vi "Set Timing.vi"(8 "error in (no error)":errorcluster, 9 "Timing Engine":T1=enum."Low Speed", 10 "TimingCfg":T2, 11 "Chassis Cfg":refnum<class "ChassisCfg.lvclass">) -> (0 "error out":errorcluster, 3 "Chassis Cfg":refnum<class "ChassisCfg.lvclass">)   [LabVIEW 2018, in "Configuration Grandmaster.lvlib" / "ChassisCfg.lvclass"]
uses:
  ChassisCfg.lvclass
  Common/Controls/Group Timing Info.ctl
  Common/Controls/TE_Designator.ctl
  ChassisCfg.lvclass/ChassisCfg.ctl
  Class Timing Group/TimingGrp.lvclass
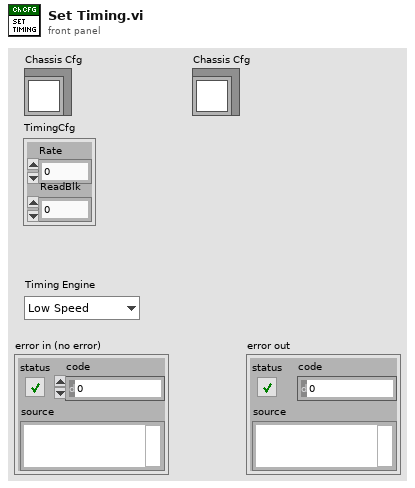
[diagram p1: front panel]
types:
  T1 = typedef "TE_Designator.ctl" = enum16{"High Speed", "Low Speed"}
  T2 = typedef "Group Timing Info.ctl" = cluster{"Rate":dbl, "ReadBlk":i32}
  T3 = typedef "LS Lock Sizes.ctl" = enum16{"No", "250ms", "500ms", "1s"}
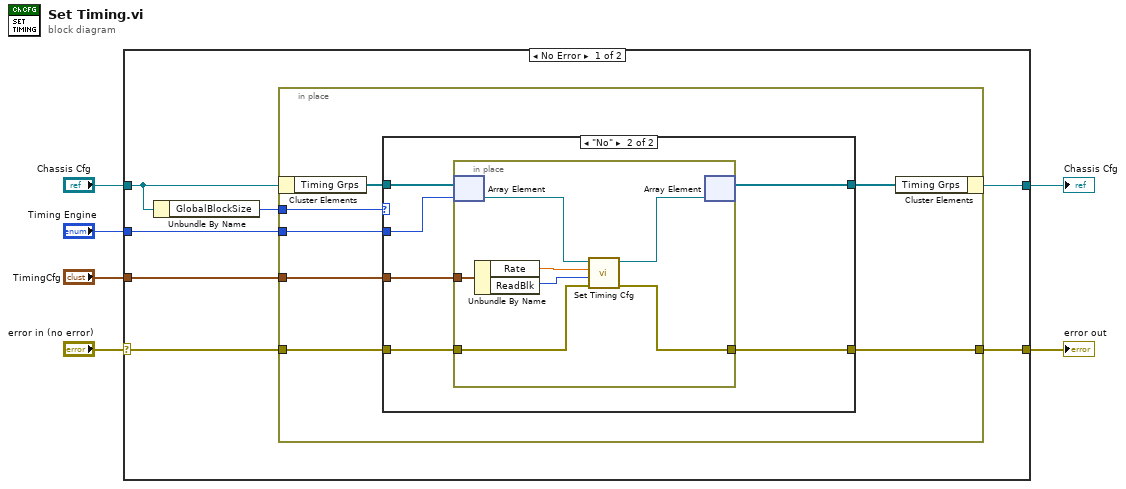
[diagram p0: block diagram]
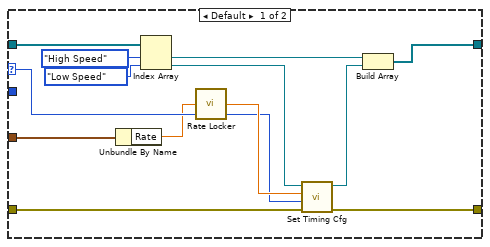
[diagram p2: hidden frame]
diagram:
  n1 = case shown="No Error" "error in (no error)" {
    selector: "error in (no error)" -> [w7 w48]
    tunnel: "TimingCfg" -> [w13 _]
    tunnel: "Timing Engine" -> [w12 _]
    tunnel: [w11 w48] -> w4
    tunnel: [w10 w49] -> w3
    tunnel: "Chassis Cfg" -> [w9 w49]
    frame No Error {
      n2 = Unbundle By Name(w9) -> ("GlobalBlockSize"=w8:T3)
      n3 = in-place {
        in-place-border: w7 -> [w20]
        in-place-border: w13 -> [w19]
        in-place-border: w12 -> [w18]
        in-place-border: [w17] -> w11
        in-place-border: w8 -> [w14]
        n4 = in-place-cluster #1(w9) -> ("Timing Grps"=w16:refnum<class "TimingGrp.lvclass">[])
        n5 = case shown="\"No\"" w14 {
          selector: w14 -> [w33 _]
          tunnel: w19 -> [w34 w39]
          tunnel: w20 -> [w31 w40]
          tunnel: [w21 w38] -> w17
          tunnel: [w28 w35] -> w15
          tunnel: w16 -> [w25 w36]
          tunnel: w18 -> [_ w37]
          frame Default {
            n6 = Unbundle By Name(w34) -> ("Rate"=w32:dbl)
            n7 = Index Array(array=w25, index #1=TE_Designator."High Speed" ("Timing Engine"), index #2=TE_Designator."Low Speed" ("Timing Engine")) -> (element #1=w23:refnum<class "TimingGrp.lvclass">, element #2=w24:refnum<class "TimingGrp.lvclass">)
            n8 = call "Rate Locker.vi"("LockToLS"=w33, "LSCfg.Rate"=w32) -> ("LSCfg.ReadBlk"=w29:i32, "LSCfg.Rate"=w30:dbl)  [unwired: 1 in, 1 out]
            n9 = call "Set Timing Cfg.vi"("error in"=w31, "ReadBlk"=w29, "Rate"=w30, "TimingGrp in"=w24) -> ("error out"=w21:errorcluster, "TimingGrp in"=w22:refnum<class "TimingGrp.lvclass">)  [unwired: 6 in]
            n10 = Build Array(w23, w22) -> (w28:refnum<class "TimingGrp.lvclass">[])
          }
          frame "No" {
            n11 = in-place {
              in-place-border: w40 -> [w47]
              in-place-border: w39 -> [w46]
              in-place-border: [w41] -> w38
              n12 = in-place-array #2(w36, w37) -> (w43:refnum<class "TimingGrp.lvclass">)
              n13 = Unbundle By Name(w46) -> ("Rate"=w45:dbl, "ReadBlk"=w44:i32)
              n14 = call "Set Timing Cfg.vi"("error in"=w47, "ReadBlk"=w44, "Rate"=w45, "TimingGrp in"=w43) -> ("error out"=w41:errorcluster, "TimingGrp in"=w42:refnum<class "TimingGrp.lvclass">)  [unwired: 6 in]
              n15 = in-place-array #2(w42) -> (w35:refnum<class "TimingGrp.lvclass">[])  [unwired: 1 out]
            }
          }
        }
        n16 = in-place-cluster #1("Timing Grps"=w15) -> (w10:refnum<class "ChassisCfg.lvclass">)
      }
    }
    frame Error {
    }
  }
  "Chassis Cfg" <- w3
  "error out" <- w4
